vi "Set DDG Lite Inter Pulse Delay.vi"(10 "fDelay":sgl, 11 "channel":u32(ring)=65535 items=["AT_DDGLite_ChannelA"=1073741824, "AT_DDGLite_ChannelB"=1073741825, "AT_DDGLite_ChannelC"=1073741826]) -> (3 "function return":u32)   [LabVIEW 2018, in "Copy of Andor SDK.lvlib"]
doc: "EXPNETTYPE unsigned int WINAPI SetDDGLiteInterPulseDelay(AT_DDGLiteChannelId channel, float fDelay);"
uses:
  Copy of Andor SDK.lvlib
  <userlib>/Andor SDK/ATMCD32D.dll
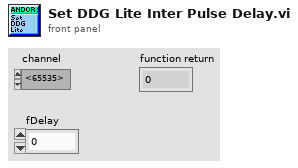
[diagram p1: front panel]
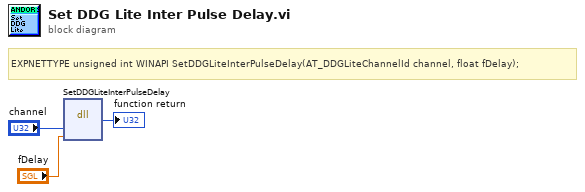
[diagram p0: block diagram]
diagram:
  # "EXPNETTYPE unsigned int WINAPI SetDDGLiteInterPulseDelay(AT_DDGLiteChannelId channel, float fDelay);"
  n1 = dll-call lib="C:/Program Files (x86)/National Instruments/LabVIEW 2018/user.lib/Andor SDK/ATMCD32D.*" fn="SetDDGLiteInterPulseDelay"("channel"="channel", "fDelay"="fDelay") -> (→"function return":u32)  [unwired: 5 in, 2 out]
